vi "CleanupLogDirectory.vi"(0 "BuffersIn":T1={"Channels"=[], "PosttriggerBuffer"=refnum, "PretriggerBuffer"=refnum, "BlockSizePerChannel"=0, " logging semaphore"=refnum, "Log refnum"=refnum, "snapshotBuffer"=refnum, "logDirectory"=path "", "logPrefix"="", "decimation factor"=1, "max files"=0, "SampleRate"=0.0}, 11 "error in":errorcluster) -> (4 "BuffersOut":T1={"Channels"=[], "PosttriggerBuffer"=refnum, "PretriggerBuffer"=refnum, "BlockSizePerChannel"=0, " logging semaphore"=refnum, "Log refnum"=refnum, "snapshotBuffer"=refnum, "logDirectory"=path "", "logPrefix"="", "decimation factor"=1, "max files"=0, "SampleRate"=0.0}, 15 "error out":errorcluster)   [LabVIEW 2015, in "BufferLogging.lvlib"]
uses:
  BufferLogging.lvlib
  Buffers.ctl
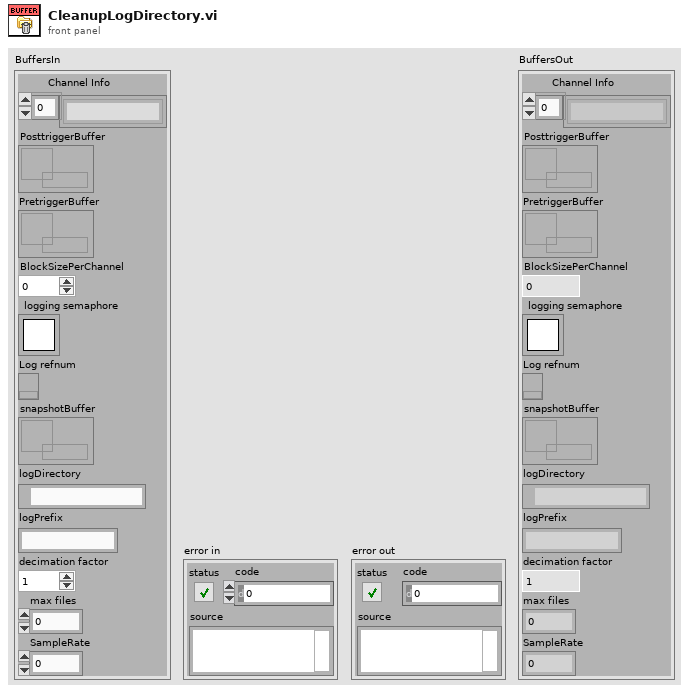
[diagram p1: front panel]
types:
  T1 = typedef "BufferLogging.lvlib/Buffers.ctl" = cluster{"Channels":string[], "PosttriggerBuffer":refnum<queue>, "PretriggerBuffer":refnum<queue>, "BlockSizePerChannel":i32, " logging semaphore":T2, "Log refnum":refnum<k34>, "snapshotBuffer":refnum<data-value>, "logDirectory":path, "logPrefix":string, "decimation factor":i32, "max files":i32, "SampleRate":dbl}
  T2 = typedef "Semaphore RefNum" = refnum<k1>
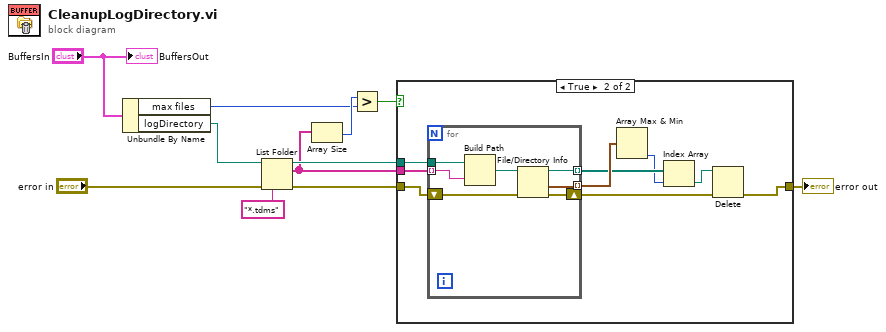
[diagram p0: block diagram]
diagram:
  n1 = Unbundle By Name("BuffersIn") -> ("max files"=w4:i32, "logDirectory"=w3:path)
  n2 = List Folder(path=w3, pattern="*.tdms", error in="error in") -> (path out=w10:path, filenames=w7:string[], error out=w6:errorcluster)  [unwired: 1 in, 1 out]
  n3 = Array Size(array=w7) -> (size(s)=w9:i32)
  n4 = Greater?(x=w9, y=w4) -> (0:w8:bool)
  n5 = case shown="True" w8 {
    tunnel: w10 -> [_ w21]
    tunnel: w7 -> [_ w20]
    tunnel: w6 -> [w12 w19]
    tunnel: [w12 w13] -> w1
    frame False {
    }
    frame True {
      n6 = for {
        tunnel: w21 -> [w28]
        tunnel: w20 -> [w27] mode=indexing
        shift-right: [w24] -> w15
        shift-left: w19 -> [w25]
        tunnel: [w23] -> w18 mode=indexing
        tunnel: [w22] -> w17 mode=indexing
        n7 = Build Path(base path=w28, name or relative path=w27) -> (appended path=w26:path)
        n8 = File/Directory Info(path=w26, error in=w25) -> (path out=w22:path, last mod=w23:timestamp, error out=w24:errorcluster)  [unwired: 4 out]
      }
      n9 = Array Max & Min(array=w18) -> (min index (indices)=w16:i32)  [unwired: 3 out]
      n10 = Index Array(array=w17, index=w16) -> (element=w14:path)
      n11 = Delete(path (use dialog)=w14, error in=w15) -> (error out=w13:errorcluster)  [unwired: 3 in, 2 out]
    }
  }
  "error out" <- w1
  "BuffersOut" <- "BuffersIn"
